vi "Strings und Zeitstempel verknuepfen v2.vi"(8 "String 2 hinzufügen":string, 9 "String 1 hinzufügen":string, 11 "Eingangs String":string) -> (2 "Verknüpfter String":string)   [LabVIEW 2020, in "allgemeine Sub-VIs.lvlib"]
uses:
  allgemeine Sub-VIs.lvlib
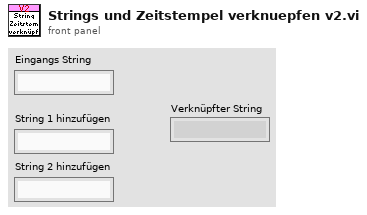
[diagram p1: front panel]
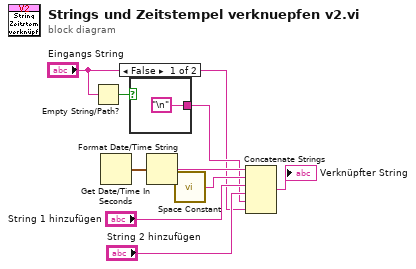
[diagram p0: block diagram]
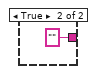
[diagram p2: hidden frame]
diagram:
  n1 = Empty String/Path?(string/path="Eingangs String") -> (empty?=w9:bool)
  n2 = Get Date/Time In Seconds() -> (seconds since 1Jan1904=w8:timestamp)
  n3 = case shown="False" w9 {
    tunnel: ["\n" ""] -> w2
    frame False {
    }
    frame True {
    }
  }
  n4 = Format Date/Time String(seconds (now)=w8) -> (date/time string=w7:string)  [unwired: 2 in]
  n5 = call <vilib>:"Space Constant.vi"() -> ("String"=w6:string)
  n6 = Concatenate Strings(w7, w6, "String 1 hinzufügen", "String 2 hinzufügen", w2, "Eingangs String") -> (→"Verknüpfter String":string)
